vi "查询.vi"(10 "点":cluster{"x":dbl, "y":dbl}={"x"=1.0, "y"=10.0}, 11 "地图":u32[][](array[colorbox])) -> (3 "索引1":enum16{"空白", "蛇", "食物", "墙", "传送门"}(ring))   [LabVIEW 2012]
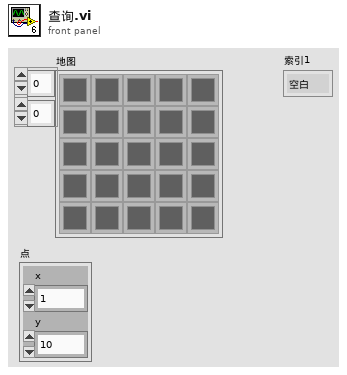
[diagram p1: front panel]
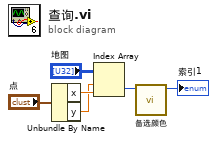
[diagram p0: block diagram]
diagram:
  n1 = Unbundle By Name("点") -> ("x"=w4:dbl, "y"=w3:dbl)
  n2 = Index Array(array="地图", index (row)=w3, index (col)=w4) -> (element=w2:u32)
  n3 = call "备选颜色.vi"("颜色1"=w2) -> ("索引1"=→"索引1":enum16{"空白", "蛇", "食物", "墙", "传送门"})  [unwired: 9 in, 1 out]
